vi "Set Output.vi"(8 "error in":errorcluster, 10 "Output":bool, 11 "Power Supply in":refnum<class "Power Supply.lvclass">) -> (0 "error out":errorcluster, 3 "Power Supply out":refnum<class "Power Supply.lvclass">)   [LabVIEW 2018, in "Power Supply.lvlib" / "Power Supply.lvclass"]
doc: "This VI stores the output state setting and sends all updated settings to the power supply."
uses:
  Power Supply.lvclass
  Power Supply.lvclass/Power Supply.ctl
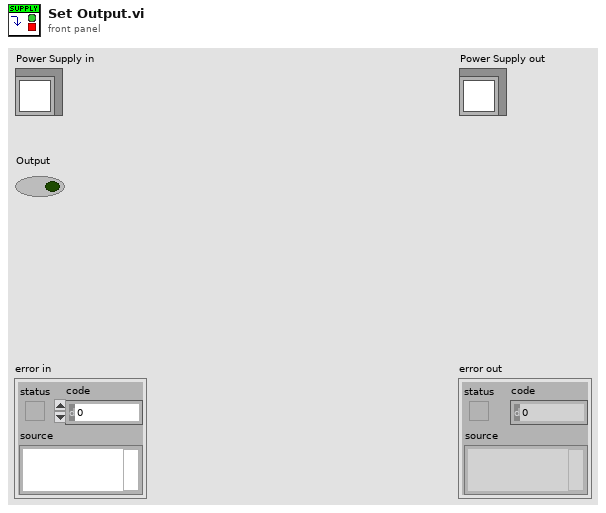
[diagram p1: front panel]
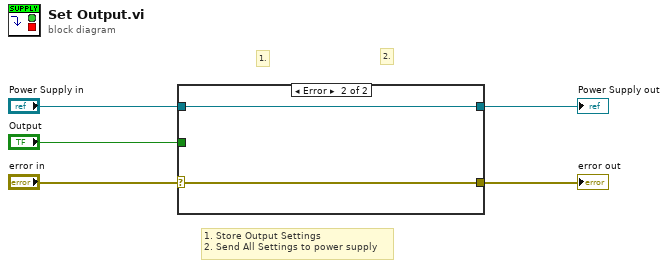
[diagram p0: block diagram]
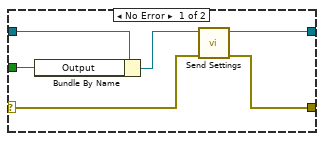
[diagram p2: hidden frame]
diagram:
  # "2."
  # "1."
  # "1. Store Output Settings\n2. Send All Settings to power supply"
  n1 = case shown="Error" "error in" {
    selector: "error in" -> [w6 w13]
    tunnel: [w11 w13] -> w5
    tunnel: "Power Supply in" -> [w10 w12]
    tunnel: [w9 w12] -> w3
    tunnel: "Output" -> [w8 _]
    frame No Error {
      n2 = Bundle By Name(cluster=w10, "Output"=w8) -> (w7:refnum<class "Power Supply.lvclass">)
      n3 = call-dynamic "Send Settings.vi"("error in (no error)"=w6, "Power Supply in"=w7) -> ("error out"=w11:errorcluster, "Power Supply out"=w9:refnum<class "Power Supply.lvclass">)  [unwired: 8 in]
    }
    frame Error {
    }
  }
  "error out" <- w5
  "Power Supply out" <- w3
